vi "observacao_0MQ.vi"() -> ()   [LabVIEW 2012, in "Shared_160.lvlib"] (continued)
            # "MUDANÇA 10/8/2010 \nIncluídos:\n- Nome do instrumento\n- RA do telescópio"
            # "OBS: O Arquivo é inicialmente apagado para \nEvitar que fique corrompido!"
            # "Escreve arquivo com Dados para o Uso da Página do PDA"
            n1086 = global read "Global_Telescopio.vi" "Lista Instrumentos"() -> (w1420:string[])
            n1087 = global read "Global_Telescopio.vi" "Sideral Time"() -> (w1410:dbl)
            n1088 = global read "Global_Telescopio.vi" "PosAH"() -> (w1411:dbl)
            n1089 = global read "Global_Telescopio.vi" "Instrum"() -> (w1419:u16)
            n1090 = local read "DOMO_ENC"() -> (w1432:string)
            n1091 = local read "CUP_STAT"() -> (w1428:string)
            n1092 = local read "AH_STAT"() -> (w1430:string)
            n1093 = local read "Sideral time"() -> (w1439:string)
            n1094 = local read "AH_ENC"() -> (w1434:string)
            n1095 = local read "UT"() -> (w1438:string)
            n1096 = Subtract(x=w1410, y=w1411) -> (x-y=w1415:dbl)
            n1097 = Add(x=6.283185307179586, y=w1415) -> (x+y=w1414:dbl)
            n1098 = Less Than 0?(x=w1415) -> (x < 0?=w1412:bool)
            n1099 = call "Retira_tudo_depois_da_virgula.vi"("Entrada"=w1439) -> ("Saída"=w1436:string)
            n1100 = local read "TUBO_STAT"() -> (w1427:string)
            n1101 = Format Date/Time String(time format string (%c)="%H:%M:%S") -> (date/time string=w1422:string)  [unwired: 2 in]
            n1102 = local read "FOCO_ENC"() -> (w1431:string)
            n1103 = local read "DEC_STAT"() -> (w1429:string)
            n1104 = local read "DEC_ENC"() -> (w1433:string)
            n1105 = Select(t=w1414, s=w1412, f=w1415) -> (s? t:f=w1416:dbl)
            n1106 = Index Array(array=w1420, index=w1419) -> (element=w1421:string)
            n1107 = Format Date/Time String(time format string (%c)="%d/%m/%Y") -> (date/time string=w1423:string)  [unwired: 2 in]
            n1108 = call "Retira_tudo_depois_da_virgula.vi"("Entrada"=w1438) -> ("Saída"=w1435:string)
            n1109 = call <vilib>:"Trim Whitespace.vi"("string"=w1436) -> ("trimmed string"=w1426:string)  [unwired: 1 in]
            n1110 = call "rad_hms.vi"("TRUE=HORA\nFALSE=GRAU"=TRUE, "Radiano"=w1416) -> ("Hora/Graus Texto Decimal"=w1409:string)  [unwired: 3 in]
            n1111 = String To Path(string="C:\\TCS\\ARQUIVOS\\DadosTCSPD.txt") -> (path=w1440:path)
            n1112 = Concatenate Strings(w1423, w1418, w1422, w1418, w1435, w1418, w1426, w1418, w1434, w1418, w1433, w1418, w1432, w1418, w1431, w1418, w1430, w1418, w1429, w1418, w1428, w1418, w1427, w1418, w1421, w1418, w1409, w1418) -> (w1442:string)
            n1113 = case shown="True" "Case Constant\n(See Context Help) 2" {
              tunnel: [w1451 w1454] -> w1441
              tunnel: w1440 -> [w1451 w1453]
              frame False {
              }
              frame True {
                n1114 = Delete(path (use dialog)=w1453) -> (deleted path=w1454:path, error out=→"error out":errorcluster)  [unwired: 4 in, 1 out]
              }
            }
            n1115 = call <vilib>:"Open_Create_Replace File.vi"("function (open:0)"=T8."open or create", "file path"=w1441) -> ("error out"=w1446:errorcluster, "refnum"=w1449:refnum<file>)  [unwired: 6 in, 2 out]
            n1116 = Set File Position(refnum=w1449, from (0:start)=enum16{"start", "end", "current"}."start" ("pos mode (0:2)"), error in=w1446) -> (refnum out=w1408:refnum<file>, error out=w1407:errorcluster)  [unwired: 1 in]
            n1117 = Write to Binary File(file (use dialog)=w1408, data=w1442, error in=w1407, 5:FALSE ("prepend array or string size? (T)")) -> (refnum out=w1448:refnum<file>, error out=w1447:errorcluster)  [unwired: 2 in, 1 out]
            n1118 = Close File(refnum=w1448, error in=w1447) -> (error out=w1450:errorcluster)  [unwired: 1 out]
            n1119 = call <vilib>:"Simple Error Handler.vi"("error in (no error)"=w1450) -> ()  [unwired: 4 in, 5 out]
          }
          frame #15 {
            # "Página do PDA"
            # "http://192.168.1.1:1080/pdaWeb/"
            # "TRATAMENTO DO PDA"
            n1120 = stacked-sequence {
              frame #0 {
                # "MUDANÇA  3/9/2010 \nIncluído case abaixo e código de seu estado TRUE para apagar eventuais comandos do PDA enviados antes do TCSPD rodar."
                n1121 = First Call?() -> (First Call?: T/F=w1455:bool)
                n1122 = case shown="True" w1455 {
                  frame False {
                    # "MUDANÇA  4/9/2010 \nSubstituída a VI \"New Read PPC\" pela \"Trata PDA\" a qual evita que o telescópio seja apontado para regiões proibidas (inclinação excessiva)."
                    # "lê e interpreta o arquivo ppc.txt"
                    n1123 = call "Trata PDA.vi"() -> ()  [unwired: 2 in]
                  }
                  frame True {
                    n1124 = call "Find ppctxt.vi"() -> ("Existe ppc.txt?"=w1457:bool, "ppc.txt Path"=w1456:path)  [unwired: 1 in]
                    n1125 = case shown="True" w1457 {
                      tunnel: w1456 -> [_ w1458]
                      frame False {
                      }
                      frame True {
                        # "limpa o arquivo ppc.txt"
                        n1126 = call "Wipe file.vi"("ppc path"=w1458) -> ()  [unwired: 2 out]
                      }
                    }
                  }
                }
              }
              frame #1 {
                n1127 = case shown="False" "Case Constant\n(See Context Help) 3" {
                  frame False {
                  }
                  frame True {
                    # "MUDANÇA:\nÉ necesário \nsubstituir as variáveis simuladas pelas do Sistema"
                    # "Simula os dados sendo alterados pela\nmovimentação do sistema"
                    n1128 = call "Data Table.vi"() -> ()  [unwired: 1 in]
                  }
                }
              }
              frame #2 {
                n1129 = case shown="True" "Case Constant\n(See Context Help) 4" {
                  frame False {
                  }
                  frame True {
                    # "Lê o arquivo padrão para o equip/o\nselecionado pelo PDA e grava o\narquivo ppcDisplay.htm adequado"
                    n1130 = call "Update Frame.vi"() -> ("Timeout"=w1461:u32)  [unwired: 2 in, 3 out]
                    n1131 = Wait Until Next ms Multiple(millisecond multiple=w1461) -> ()  [unwired: 1 out]
                  }
                }
              }
            }
          }
        }
        n1132 = global read "Global_Telescopio.vi" "Flag-Rotator"() -> (w77:bool)
        n1133 = case shown="True" w77 {
          frame False {
          }
          frame True {
            n1134 = local write "Setup, Pointing & Guiding"(T2."ROTATOR" ("Setup, Pointing & Guiding")) -> ()
          }
        }
      }
      frame #2 {
        n1135 = case shown="\"UTILS \"" "Setup, Pointing & Guiding" {
          frame "POINTING", Default {
            n1136 = stacked-sequence {
              frame #0 {
                # "Clear Dados"
                n1137 = local read "ChkCalLocal"() -> (w1463:bool)
                n1138 = case shown="False" w1463 {
                  selector: w1463 -> [w1465 _]
                  frame False {
                    # "Para de Piscar/Blink\no botão"
                    n1139 = property on="ChkCalLocal" class="Bool (strict)"("Blinking"=w1465) -> ()  [unwired: 2 in, 2 out]
                  }
                  frame True {
                  }
                }
                n1140 = case shown="True" "BtPointObjClear" {
                  frame False {
                  }
                  frame True {
                    w1466 = ""
                    n1141 = local write "StrPointObjName"(w1466) -> ()
                    n1142 = local write "StrPointObjPMRA"(w1466) -> ()
                    n1143 = local write "StrPointObjPMDEC"(w1466) -> ()
                    n1144 = local write "StrPointObjRA"(w1466) -> ()
                    n1145 = local write "StrPointObjDEC"(w1466) -> ()
                    n1146 = local write "StrPointObjEpoch"(w1466) -> ()
                    n1147 = local write "StrPointTargetRA"(w1466) -> ()
                    n1148 = local write "StrPointTargetDEC"(w1466) -> ()
                  }
                }
              }
              frame #1 {
                w1473 = ""
                # "A forma como os mostradores da janela TARGET são carregados está indefinida.\nVamos colocar um botão SET ao lado do botão CLEAR na janela OBJECT.\nQuando o botão SET for pressionado, os mostradores da janela TARGET\nseriam calculados a partir dos valores da janela OBJECT."
                n1149 = local read "StrPointObjDEC"() -> (w1474:string)
                n1150 = local read "StrPointObjRA"() -> (w1475:string)
                n1151 = local read "StrPointObjPMDEC"() -> (w1467:string)
                n1152 = local read "StrPointObjPMRA"() -> (w1468:string)
                n1153 = Not Equal?(x=w1475, y=w1473) -> (x != y?=w1472:bool)
                n1154 = Not Equal?(x=w1474, y=w1473) -> (x != y?=w1471:bool)
                n1155 = local read "pressão atm"() -> (w1477:string)
                n1156 = local read "Temp amb"() -> (w1478:string)
                n1157 = local read "hum local"() -> (w1476:string)
                n1158 = And(x=w1472, y=w1471) -> (x .and. y?=w1469:bool)
                n1159 = And(x="BtPointPrecess", y=w1469) -> (x .and. y?=w1470:bool)
                n1160 = case shown="True" w1470 {
                  tunnel: w1475 -> [_ w1486]
                  tunnel: w1474 -> [_ w1485]
                  tunnel: w1478 -> [_ w1484]
                  tunnel: w1477 -> [_ w1483]
                  tunnel: w1476 -> [_ w1482]
                  tunnel: w1468 -> [_ w1481]
                  tunnel: w1467 -> [_ w1480]
                  frame False {
                  }
                  frame True {
                    n1161 = stacked-sequence {
                      tunnel: w1486 -> [w1520 _ _]
                      tunnel: w1485 -> [w1518 _ _]
                      tunnel: w1484 -> [w1528 _ _]
                      tunnel: w1483 -> [w1527 _ _]
                      tunnel: w1482 -> [w1526 _ _]
                      tunnel: w1481 -> [w1494 _ _]
                      tunnel: w1480 -> [w1493 _ _]
                      frame #0 {
                        # "PROCESSO PRECESSÃO"
                        # "MUDANÇA:\nVI Botao SET trocada por Botao Precess, eliminando entrada do Frame de coord. (Mean, Topo, Geo)"
                        n1162 = local read "ChkPointPrecessed"() -> (w1498:bool)
                        n1163 = call "Comma_to_Point.vi"("Lat_A"=w1518) -> ("Saída"=w1513:string)
                        n1164 = call "Comma_to_Point.vi"("Lat_A"=w1520) -> ("Saída"=w1516:string)
                        n1165 = call "hms_rad.vi"("True = hora"=FALSE, "Texto Graus"=w1513) -> ("radianos"=w1512:dbl)  [unwired: 3 in]
                        n1166 = call "hms_rad.vi"("True = hora"=TRUE, "Texto Graus"=w1516) -> ("radianos"=w1515:dbl)  [unwired: 3 in]
                        n1167 = call "Comma_to_Point.vi"("Lat_A"=w1527) -> ("Saída"=w1496:string)
                        n1168 = call "Comma_to_Point.vi"("Lat_A"=w1526) -> ("Saída"=w1495:string)
                        n1169 = call "Comma_to_Point.vi"("Lat_A"=w1528) -> ("Saída"=w1497:string)
                        n1170 = call "Arcsec to Rad_ String.vi"("VAR ARCSEC"=w1494) -> ("VAR RAD"=w1492:string)
                        n1171 = Number To Fractional String(use system decimal point (T)=FALSE, number=w1512, precision (6)=i16 9) -> (F-format string=w1501:string)  [unwired: 1 in]
                        n1172 = Number To Fractional String(use system decimal point (T)=FALSE, number=w1515, precision (6)=i16 9) -> (F-format string=w1502:string)  [unwired: 1 in]
                        n1173 = call "Arcsec to Rad_ String.vi"("VAR ARCSEC"=w1493) -> ("VAR RAD"=w1491:string)
                        n1174 = call "Botão Precess.vi"("AR"=w1502, "Precessed Coord."=w1498, "Dec"=w1501, "Temp local amb(K)"=w1497, "Pressao atm local (mB)"=w1496, "Hum rel local"=w1495, "Var RA"=w1492, "Var DEC"=w1491) -> ("RA"=w1530:dbl, "DEC"=w1487:dbl, "Hora Sideral (rad)"=w1529:dbl, "Dist. Zenital (rad)"=w1500:dbl, "Observed HA (radians)"=→"HA obs":dbl, "Massa de Ar"=w1499:dbl)  [unwired: 2 in]
                        "RA obs" <- w1530
                        "DEC obs" <- w1487
                        n1175 = local write "Zenital angle"(w1500) -> ()
                        n1176 = call "rad_hms.vi"("TRUE=HORA\nFALSE=GRAU"=FALSE ("TRUE=HORA\nFALSE=GRAU"), "Radiano"=w1487) -> ("Hora/Graus Texto Decimal"=w1508:string)  [unwired: 3 in]
                        n1177 = call "rad-graus.vi"("Radiano"=w1500) -> ("Graus"=w1525:dbl)
                        n1178 = Number To Fractional String(number=w1499, precision (6)=i16 3) -> (F-format string=→"Air Mass":string)  [unwired: 2 in]
                        n1179 = Number To Fractional String(number=w1525, precision (6)=i16 1) -> (F-format string=→"Zenital Angle":string)  [unwired: 2 in]
                        n1180 = call "rad_hms.vi"("TRUE=HORA\nFALSE=GRAU"=TRUE ("TRUE=HORA"), "Radiano"=w1530) -> ("Hora/Graus Texto Decimal"=w1510:string)  [unwired: 3 in]
                        n1181 = local write "StrPointTargetDEC"(w1508) -> ()
                        n1182 = local write "StrPointTargetRA"(w1510) -> ()
                        n1183 = disable-structure shown="Disabled" {
                          disable-tunnel: [w1534 _] -> _
                          disable-tunnel: w1530 -> [w1533 _]
                          disable-tunnel: w1529 -> [w1532 _]
                          disable-tunnel: w1487 -> [w1531 _]
                          frame Disabled {
                            n1184 = call "Hora_Limite.vi"("Asc Reta RA rad"=w1533, "Sideral Time rad"=w1532, "Declinação rad"=w1531) -> ("TO Tempo de Observação Horas"=w1534:dbl)  [unwired: 2 in]
                          }
                          frame Enabled {
                          }
                        }
                        n1185 = call "Novo_tempo_obs_inicial.vi"("TS"=w1529, "RA"=w1530, "DEC"=w1487) -> ("TO rad"=w1488:dbl)  [unwired: 7 in, 1 out]
                        n1186 = case shown="True" "TRUE=HORA\nFALSE=GRAU" {
                          frame False {
                          }
                          frame True {
                            # "Sincroniza hora do\nPC com GPS"
                            n1187 = call "About_Time.vi"() -> ()  [unwired: 1 in]
                          }
                        }
                        n1188 = call "rad_hms.vi"("TRUE=HORA\nFALSE=GRAU"=TRUE ("TRUE=HORA\nFALSE=GRAU"), "Radiano"=w1488) -> ("Hora/Graus Texto Decimal"=→"Tempo Obs":string)  [unwired: 3 in]
                      }
                      frame #1 {
                        # "Testa o ângulo zenital menor que 70º o led \"Working Area\" \naceso na cor verde se o ângulozenital menor que 70º e \nvermelho em caso cont rário."
                        n1189 = global read "Global_Telescopio.vi" "Piscar working area"() -> (w1541:bool)
                        n1190 = global read "Global_Telescopio.vi" "working area = VERDE"() -> (w1540:bool)
                        n1191 = global read "Global_Telescopio.vi" "ativar botão GO"() -> (w1538:bool)
                        n1192 = case shown="True" w1540 {
                          frame False {
                            # "False=Vermelho"
                            n1193 = local write "LedPointWorkArea"(FALSE ("LedPointWorkArea")) -> ()
                          }
                          frame True {
                            # "True=Verde"
                            "LedPointWorkArea" <- TRUE ("LedPointWorkArea")
                          }
                        }
                        n1194 = global write "Global_Telescopio.vi" "Botão GO = STOP"(FALSE ("Botão GO = STOP")) -> ()
                        n1195 = case shown="True" w1538 {
                          selector: w1538 -> [_ w1542]
                          frame False {
                          }
                          frame True {
                            n1196 = property on="BtTargetPoint" class="Bool"("Visible"=w1542) -> ()  [unwired: 2 in, 2 out]
                          }
                        }
                        n1197 = global write "Global_Telescopio.vi" "Piscar working area"(w1541) -> ()
                        n1198 = global read "Global_Telescopio.vi" "desativar botão GO"() -> (w1539:bool)
                        n1199 = case shown="True" w1539 {
                          selector: w1539 -> [_ w1544]
                          frame False {
                          }
                          frame True {
                            n1200 = Not(x=w1544) -> (.not. x?=w1543:bool)
                            n1201 = property on="BtTargetPoint" class="Bool"("Visible"=w1543) -> ()  [unwired: 2 in, 2 out]
                          }
                        }
                        n1202 = property on="LedPointWorkArea" class="Bool (strict)"("Visible"=TRUE ("Botão GO = STOP")) -> ()  [unwired: 2 in, 2 out]
                        n1203 = property on="LedPointing" class="Bool (strict)"("Visible"=FALSE) -> ()  [unwired: 2 in, 2 out]
                      }
                      frame #2 {
                        n1204 = global read "Global_Telescopio.vi" "CalDEC Local"() -> (w1552:dbl)
                        n1205 = global read "Global_Telescopio.vi" "CalAH Local"() -> (w1553:dbl)
                        n1206 = local read "ChkCalLocal"() -> (w1547:bool)
                        n1207 = Not Equal To 0?(x=w1553) -> (x != 0?=w1550:bool)
                        n1208 = Not Equal To 0?(x=w1552) -> (x != 0?=w1551:bool)
                        n1209 = Or(x=w1550, y=w1551) -> (x .or. y?=w1548:bool)
                        n1210 = And(x=w1547, y=w1548) -> (x .and. y?=w1549:bool)
                        n1211 = case shown="True" w1549 {
                          frame False {
                          }
                          frame True {
                            n1212 = local read "HA obs"() -> (w1573:dbl)
                            n1213 = local read "DEC obs"() -> (w1567:dbl)
                            n1214 = global read "Global_Telescopio.vi" "AH Zero Local"() -> (w1571:dbl)
                            n1215 = global read "Global_Telescopio.vi" "DEC Zero Local"() -> (w1566:dbl)
                            n1216 = global read "Global_Telescopio.vi" "Raio Máximo"() -> (w1555:dbl)
                            n1217 = Cosine(x=w1567) -> (cos(x)=w1572:dbl)
                            n1218 = Cosine(x=w1566) -> (cos(x)=w1570:dbl)
                            n1219 = Multiply(x=w1573, y=w1572) -> (x*y=w1569:dbl)
                            n1220 = Multiply(x=w1571, y=w1570) -> (x*y=w1568:dbl)
                            n1221 = Subtract(x=w1567, y=w1566) -> (x-y=w1562:dbl)
                            n1222 = Multiply(x=w1562, y=w1562) -> (x*y=w1565:dbl)
                            n1223 = Subtract(x=w1569, y=w1568) -> (x-y=w1561:dbl)
                            n1224 = Multiply(x=w1561, y=w1561) -> (x*y=w1563:dbl)
                            n1225 = Add(x=w1563, y=w1565) -> (x+y=w1564:dbl)
                            n1226 = Square Root(x=w1564) -> (sqrt(x)=w1560:dbl)
                            n1227 = Multiply(x=w1560, y=180.0) -> (x*y=w1558:dbl)
                            n1228 = Divide(x=w1558, y=3.141592653589793) -> (x/y=w1556:dbl)
                            n1229 = Greater?(x=w1556, y=w1555) -> (0:w1554:bool)
                            n1230 = property on="ChkCalLocal" class="Bool (strict)"("Blinking"=w1554) -> ()  [unwired: 2 in, 2 out]
                          }
                        }
                      }
                    }
                  }
                }
              }
              frame #2 {
                # "Clicando-se essa Tecla\nInicia-se o Apontamento"
                n1231 = local read "hum local"() -> (w1582:string)
                n1232 = local read "StrPointObjRA"() -> (w1584:string)
                n1233 = local read "StrPointObjDEC"() -> (w1583:string)
                n1234 = local read "StrPointObjPMDEC"() -> (w1575:string)
                n1235 = local read "pressão atm"() -> (w1576:string)
                n1236 = local read "StrPointObjPMRA"() -> (w1574:string)
                n1237 = local read "Temp amb"() -> (w1577:string)
                n1238 = control-ref of="BtTargetPoint"() -> (w1579:refnum<vi>)
                n1239 = property class="Bool"(reference=w1579) -> ("Boolean Text.Text"=w1580:string)  [unwired: 1 in, 2 out]
                n1240 = Equal?(x=w1580, y="POINT") -> (x = y?=w1578:bool)
                n1241 = case shown="True" "BtTargetPoint" {
                  tunnel: w1584 -> [_ w1590]
                  tunnel: w1583 -> [_ w1594]
                  tunnel: w1577 -> [_ w1591]
                  tunnel: w1576 -> [_ w1592]
                  tunnel: w1582 -> [_ w1593]
                  tunnel: w1578 -> [_ w1588]
                  tunnel: w1575 -> [_ w1587]
                  tunnel: w1574 -> [_ w1586]
                  frame False {
                  }
                  frame True {
                    n1242 = case shown="False" w1588 {
                      selector: w1588 -> [w1596 _]
                      tunnel: w1594 -> [_ w1626]
                      tunnel: w1593 -> [_ w1606]
                      tunnel: w1592 -> [_ w1605]
                      tunnel: w1591 -> [_ w1604]
                      tunnel: w1590 -> [_ w1625]
                      tunnel: w1587 -> [_ w1620]
                      tunnel: w1586 -> [_ w1621]
                      frame False {
                        w1597 = 0 ("estado")
                        # "Zera Máquina de Estado\nPelo Botão STOP"
                        n1243 = Not(x=w1596) -> (.not. x?=w1598:bool)
                        n1244 = local write "LedPointing"(w1596) -> ()
                        n1245 = global write "Global_Telescopio.vi" "Botão GO = STOP"(w1598) -> ()
                        n1246 = call "Stop.vi"() -> ()  [unwired: 1 in, 1 out]
                        n1247 = local write "statDEC"(w1597) -> ()
                        n1248 = local write "statAH"(w1597) -> ()
                        n1249 = local write "statCUP"(w1597) -> ()
                        "Flag Stop" <- TRUE ("Flag Stop")
                      }
                      frame True {
                        w1599 = ""
                        w1624 = FALSE ("use system decimal point (T)")
                        n1250 = call "Comma_to_Point.vi"("Lat_A"=w1625) -> ("Saída"=w1614:string)
                        n1251 = call "Comma_to_Point.vi"("Lat_A"=w1626) -> ("Saída"=w1615:string)
                        n1252 = call "Arcsec to Rad_ String.vi"("VAR ARCSEC"=w1621) -> ("VAR RAD"=w1602:string)
                        n1253 = call "hms_rad.vi"("True = hora"=TRUE, "Texto Graus"=w1614) -> ("radianos"=w1629:dbl)  [unwired: 3 in]
                        n1254 = call "hms_rad.vi"("True = hora"=FALSE, "Texto Graus"=w1615) -> ("radianos"=w1627:dbl)  [unwired: 3 in]
                        n1255 = call "Arcsec to Rad_ String.vi"("VAR ARCSEC"=w1620) -> ("VAR RAD"=w1603:string)
                        n1256 = local write "NAME"(w1599) -> ()
                        n1257 = local write "RA"(w1599) -> ()
                        n1258 = local write "DEC"(w1599) -> ()
                        n1259 = Number To Fractional String(use system decimal point (T)=w1624, number=w1629, precision (6)=i16 9) -> (F-format string=w1601:string)  [unwired: 1 in]
                        n1260 = Number To Fractional String(use system decimal point (T)=w1624, number=w1627, precision (6)=i16 9) -> (F-format string=w1600:string)  [unwired: 1 in]
                        n1261 = Concatenate Strings("Apontamento:" ("string"), "RA= " ("string"), w1614, " " ("string"), "DEC= " ("string"), w1615) -> ()  [unwired: 1 out]
                        n1262 = call "PrecessaoCorrigida.vi"("Coordenada do dia"="ChkPointPrecessed", "HabCorrModelo"="ChkModel", "UseLocalZero"="ChkCalLocal", "UseGlobalZero"="ChkCalGlobal", "RA"=w1601, "DEC"=w1600, "MovProprioRA"=w1602, "MovProprioDEC"=w1603, "Temp amb (K)"=w1604, "Press atm (mB)"=w1605, "Humid relat"=w1606) -> ("Estado"=w1609:i32, "RA"=w1608:dbl, "DEC"=w1607:dbl)  [unwired: 2 out]
                        n1263 = Equal To 0?(x=w1609) -> (x = 0?=w1622:bool)
                        n1264 = case shown="False" w1622 {
                          selector: w1622 -> [w1645 _]
                          tunnel: "ChkCalLocal" -> [w1657 _]
                          tunnel: "ChkCalGlobal" -> [w1656 _]
                          tunnel: w1600 -> [w1655 _]
                          tunnel: w1601 -> [w1654 _]
                          tunnel: w1603 -> [w1651 _]
                          tunnel: w1602 -> [w1650 _]
                          tunnel: w1609 -> [w1632 _]
                          tunnel: w1608 -> [w1653 _]
                          tunnel: w1607 -> [w1652 _]
                          tunnel: "ChkPointPrecessed" -> [w1648 _]
                          frame False {
                            w1635 = FALSE ("Coude")
                            w1636 = FALSE ("WeakSel")
                            w1637 = T5."Enabled" ("Disabled")
                            w1638 = TRUE ("MOUNT")
                            w1649 = 0 ("M_AH")
                            w1646 = TRUE
                            # "ABAS DE CONTROLE"
                            # "MUDANÇA:\nIncluído CASE"
                            # "Seta máquinas de\nestado aba ÚTILS"
                            n1265 = global write "Global_Telescopio.vi" "CoordDia"(w1648) -> ()
                            n1266 = global write "Global_Telescopio.vi" "CalGlobal"(w1656) -> ()
                            n1267 = global write "Global_Telescopio.vi" "CalLocal"(w1657) -> ()
                            n1268 = call "Envia LOG.vi"() -> ()  [unwired: 8 in, 2 out]
                            n1269 = global write "Global_Telescopio.vi" "TargetRA"(w1653) -> ()
                            n1270 = global write "Global_Telescopio.vi" "TargetDEC"(w1652) -> ()
                            n1271 = local write "statAH"(w1632) -> ()
                            n1272 = property on="LedPointWorkArea" class="Bool (strict)"("Visible"=FALSE ("Botão GO = STOP")) -> ()  [unwired: 2 in, 2 out]
                            n1273 = local write "statDEC"(w1632) -> ()
                            n1274 = global write "Global_Telescopio.vi" "ObjCentrado"(w1645) -> ()
                            n1275 = local write "RA on Target"(w1645) -> ()
                            n1276 = local write "DEC on Target"(w1645) -> ()
                            n1277 = local write "Dome on Target"(w1645) -> ()
                            n1278 = local read "ChkDomeEnable"() -> (w1644:bool)
                            n1279 = local write "M_AH"(w1649) -> ()
                            n1280 = local write "M_DEC"(w1649) -> ()
                            n1281 = local write "M_CUP"(w1649) -> ()
                            n1282 = case shown="True" w1644 {
                              selector: w1644 -> [w1678 _]
                              tunnel: w1632 -> [_ w1680]
                              tunnel: [0 ("Estado") w1680] -> w1643
                              tunnel: [u8 2 ("Disabled") u8 0 ("Disabled")] -> w1642
                              frame False {
                                n1283 = local write "DOME"(w1678) -> ()
                              }
                              frame True {
                              }
                            }
                            n1284 = Tick Count (ms)() -> (millisecond timer value=w1640:u32)
                            n1285 = Add(x=w1640, y=u32 120000) -> (x+y=w1641:u32)
                            n1286 = local write "Tick Cupula"(w1641) -> ()
                            n1287 = local write "GUIDER"(w1638) -> ()
                            n1288 = local write "MOUNT"(w1638) -> ()
                            n1289 = property on="LedPointing" class="Bool (strict)"("Visible"=w1646) -> ()  [unwired: 2 in, 2 out]
                            n1290 = local write "statCUP"(w1643) -> ()
                            n1291 = property on="DOME" class="Bool (strict)"("Disabled"=w1642) -> ()  [unwired: 2 in, 2 out]
                            n1292 = stacked-sequence {
                              frame #0 {
                                n1293 = local read "StrPointObjName"() -> (w1658:string)
                                n1294 = local read "StrPointObjRA"() -> (w1659:string)
                                n1295 = local read "StrPointObjDEC"() -> (w1660:string)
                                n1296 = global write "Global_Telescopio.vi" "RA AUX"(w1659) -> ()
                                n1297 = global write "Global_Telescopio.vi" "DEC AUX"(w1660) -> ()
                                n1298 = global write "Global_Telescopio.vi" "NAME OBJETO AUX"(w1658) -> ()
                              }
                              frame #1 {
                                w1662 = u16 4 items=["ZERO", "AH", "DEC", "TUBO", "CUP"] ("Controlador")
                                n1299 = call "Monta Comando.vi"("Comando"="DESLIGAR", "Dispositivo"="FLAT_WEAK", "Controlador"=w1662) -> ()  [unwired: 4 in, 3 out]
                              }
                              frame #2 {
                                w1665 = u16 4 items=["ZERO", "AH", "DEC", "TUBO", "CUP"] ("Controlador")
                                n1300 = call "Monta Comando.vi"("Comando"="DESLIGAR", "Dispositivo"="FLAT_LO", "Controlador"=w1665) -> ()  [unwired: 4 in, 3 out]
                              }
                              frame #3 {
                                w1668 = u16 4 items=["ZERO", "AH", "DEC", "TUBO", "CUP"] ("Controlador")
                                n1301 = call "Monta Comando.vi"("Comando"="DESLIGAR", "Dispositivo"="FLAT_HI", "Controlador"=w1668) -> ()  [unwired: 4 in, 3 out]
                              }
                              frame #4 {
                                w1670 = u16 4 items=["ZERO", "AH", "DEC", "TUBO", "CUP"] ("Controlador")
                                n1302 = call "Monta Comando.vi"("Comando"="DESLIGAR", "Dispositivo"="FLAT_COUDE", "Controlador"=w1670) -> ()  [unwired: 4 in, 3 out]
                              }
                              frame #5 {
                                w1673 = u16 4 items=["ZERO", "AH", "DEC", "TUBO", "CUP"] ("Controlador")
                                n1303 = call "Monta Comando.vi"("Comando"="LIGAR", "Dispositivo"="LAMP_CAM", "Controlador"=w1673) -> ()  [unwired: 4 in, 3 out]
                              }
                              frame #6 {
                                n1304 = call "Log_Apontamento.vi"() -> ()  [unwired: 12 in]
                              }
                            }
                            n1305 = local write "DOME"(FALSE ("WeakSel")) -> ()
                            n1306 = local write "WeakSel"(w1636) -> ()
                            n1307 = local write "MediumSel"(w1636) -> ()
                            n1308 = local write "StrongSel"(w1636) -> ()
                            n1309 = local write "CoudeSel"(w1636) -> ()
                            n1310 = local write "Coude"(w1635) -> ()
                            n1311 = local write "Weak"(w1635) -> ()
                            n1312 = local write "Medium"(w1635) -> ()
                            n1313 = local write "Strong"(w1635) -> ()
                            n1314 = property on="Medium" class="Bool (strict)"("Disabled"=w1637) -> ()  [unwired: 2 in, 2 out]
                            n1315 = property on="Strong" class="Bool (strict)"("Disabled"=w1637) -> ()  [unwired: 2 in, 2 out]
                            n1316 = property on="Coude" class="Bool (strict)"("DisabledEnum"=w1637) -> ()  [unwired: 2 in, 2 out]
                            n1317 = property on="Weak" class="Bool (strict)"("Disabled"=w1637) -> ()  [unwired: 2 in, 2 out]
                            "MeanDEC" <- w1655
                            "MeanRA" <- w1654
                            "LedPointing" <- w1646
                            "PM_DEC" <- w1651
                            "PM_RA" <- w1650
                            "Apontou" <- TRUE ("WeakSel")
                          }
                          frame True {
                          }
                        }
                      }
                    }
                    n1318 = property on="Delete Calagem" class="Bool"("Disabled"=u8 0) -> ()  [unwired: 2 in, 2 out]
                  }
                }
              }
              frame #3 {
                # "e o led \"Working Area\" aceso na cor verde se o ângulo\nzenital menor que 70º e vermelho em caso cont rário.\nO botão GO ao ser clicado dispara o apontamento virtual do telescópio. Caso esse\nbotão seja pressionado enquanto o led \"Working Area\" est iver vermelho, este deve\npiscar 3 vezes e nada mais é executado. Caso cont rário, o nome do botão GO passa\npara CANCEL e o led \"Mount in Posit ion\" da janela STATUS INFORMATION deve ser\ndesligado, o que provocará a simulação do apontamento do telescópio (cf. item 4.3) .\nOs valores dos comandos \"Epoch\" , \"RA Proper Mot ion\" e \"DEC Proper Mot ion\" desse\nquadro devem ser ignorados na simulação."
                # "Habilita Cancela"
                # "Habilita Apontamento"
                n1319 = case shown="True" "Case Constant\n(See Context Help) 5" {
                  frame False {
                  }
                  frame True {
                    w1686 = TRUE ("Go aux")
                    w1687 = ""
                    n1320 = local write "DEC"(w1687) -> ()
                    n1321 = local write "RA"(w1687) -> ()
                    n1322 = local write "NAME"(w1687) -> ()
                    n1323 = control-ref of="BtTargetPoint"() -> (w1688:refnum<vi>)
                    n1324 = local write "LED MOUNT"(w1686) -> ()
                    n1325 = local write "MOUNT"(w1686) -> ()
                    n1326 = property class="Bool"(reference=w1688, "Boolean Text.Text"="STOP") -> ()  [unwired: 1 in, 2 out]
                  }
                }
                n1327 = case shown="True" "Case Constant\n(See Context Help) 6" {
                  frame False {
                  }
                  frame True {
                    w1683 = FALSE ("Go aux")
                    # "Seta nome para GO"
                    n1328 = local write "LED MOUNT"(w1683) -> ()
                    n1329 = local write "MOUNT"(w1683) -> ()
                    n1330 = control-ref of="BtTargetPoint"() -> (w1684:refnum<vi>)
                    n1331 = property class="Bool"(reference=w1684, "Boolean Text.Text"="POINT") -> ()  [unwired: 1 in, 2 out]
                  }
                }
              }
              frame #4 {
                # "Detecta Edição"
                # "os valores de RA e DEC devem assumir os valores da janela OBJECT da aba POINTING ao TÉRMINO do apontamento. Durante o apontamento devem ficar apagados. Como o campo MAG daquela janela não tem um valor correspondente na janela OBJECT, o campo MAG deve ficar em branco. Apenas quando as coordenadas da janela OBJECT da aba POINTING forem preenchidos a partir do botão SET COORD da aba LIST é que o campo MAG da janela TARGET assume o valor da coluna MAG da aba LIST. Colocar um flag interno (invisível para o usuário) para definir se o campo MAG deve ou não ser preenchido com o valor da aba LIST. Quando o botão SET COORD. fosse pressionado esse flag assumiria o valor verdadeiro e caso ocorresse edição dos valores da janela \nOBJECT da aba POINTING, esse flag assumiria o valor falso e o campo MAG da janela TARGET (entre os controles das abas e as imagens) ficaria vazio durante e após o apontamento"
                n1332 = local read "StrPointObjPMRA"() -> (w1703:string)
                n1333 = local read "StrPointObjPMDEC"() -> (w1702:string)
                n1334 = local read "StrPointObjName"() -> (w1710:string)
                n1335 = local read "AUX EDITA Name"() -> (w1709:string)
                n1336 = local read "StrPointObjEpoch"() -> (w1704:string)
                n1337 = local read "AUX EDITA PMDEC"() -> (w1701:string)
                n1338 = local read "StrPointObjRA"() -> (w1708:string)
                n1339 = local read "StrPointObjDEC"() -> (w1706:string)
                n1340 = local read "AUX EDITA EPOCH"() -> (w1699:string)
                n1341 = local read "AUX EDITA PMRA"() -> (w1700:string)
                n1342 = local read "AUX EDITA DEC"() -> (w1705:string)
                n1343 = local read "AUX EDITA RA"() -> (w1707:string)
                n1344 = Not Equal?(x=w1703, y=w1700) -> (x != y?=w1694:bool)
                n1345 = Not Equal?(x=w1710, y=w1709) -> (x != y?=w1698:bool)
                n1346 = Not Equal?(x=w1704, y=w1699) -> (x != y?=w1695:bool)
                n1347 = Not Equal?(x=w1702, y=w1701) -> (x != y?=w1693:bool)
                n1348 = Not Equal?(x=w1708, y=w1707) -> (x != y?=w1697:bool)
                n1349 = Not Equal?(x=w1706, y=w1705) -> (x != y?=w1696:bool)
                n1350 = Compound Arithmetic op=OR(w1698, w1697, w1696, w1695, w1694, w1693) -> (w1690:bool)
                n1351 = local read "FLAG SET COORD"() -> (w1691:bool)
                n1352 = And(x=w1690, y=w1691) -> (x .and. y?=w1692:bool)
                n1353 = case shown="True" w1692 {
                  frame False {
                  }
                  frame True {
                    # "Se houver edição o flag é resetado"
                    n1354 = local write "MAG"("") -> ()
                    "FLAG SET COORD" <- FALSE ("FLAG SET ACOORD")
                  }
                }
              }
            }
          }
          frame "HANDSET" {
            # "PROCESSO DISPLAY DESLOCAMENTO"
            n1355 = local read "AtualDEC"() -> (w1726:dbl)
            n1356 = global read "Global_Telescopio.vi" "Sideral Time"() -> (w1719:dbl)
            n1357 = global read "Global_Telescopio.vi" "PosAH"() -> (w1717:dbl)
            n1358 = Multiply(x="Velocity (arcsec/sec)", y=100.0) -> (x*y=w1734:dbl)
            n1359 = Cosine(x=w1726) -> (cos(x)=w1725:dbl)
            n1360 = Subtract(x=w1719, y=w1717) -> (x-y=w1718:dbl)
            n1361 = Absolute Value(x=w1725) -> (abs(x)=w1722:dbl)
            n1362 = Add(x=1e-10, y=w1722) -> (x+y=w1724:dbl)
            n1363 = local read "LatchDeslocRA"() -> (w1730:dbl)
            n1364 = local read "LatchDeslocDEC"() -> (w1729:dbl)
            n1365 = global read "Global_Telescopio.vi" "PosDEC"() -> (w1720:dbl)
            n1366 = event shown="[9] \"Calagem\": Value Change" {
              selector: _ -> [_ _ _ _ _ _ _ _ _ _ _]
              dyn-events: _ -> [_ _ _ _ _ _ _ _ _ _ _]
              timeout: 10 -> [_ _ _ _ _ _ _ _ _ _ _]
              tunnel: w1734 -> [_ w1747 w1755 w1763 _ _ _ _ _ _ w1866]
              tunnel: "Global" -> [_ _ _ _ _ _ _ _ w1808 w1828 _]
              tunnel: w1718 -> [_ _ _ _ w1766 _ _ _ _ w1826 _]
              tunnel: w1720 -> [_ _ _ _ _ w1767 _ _ _ w1827 _]
              tunnel: w1724 -> [_ _ _ _ _ _ w1768 w1786 _ _ _]
              event Timeout {
                n1367 = event-data() -> ()  [unwired: 1 in, 2 out]
              }
              event "Left HS": Value Change {
                w1744 = u8 0 ("Disabled")
                n1368 = event-data() -> ("NewVal"=w1743:bool)  [unwired: 1 in, 5 out]
                "MOV_IDX_AH" <- w1743
                n1369 = call "Tx handeset.vi"("CMD On"="left" ("Comando"), "CMD Off"="stoph" ("Comando"), "Estado do Botão"=w1743, "Velocity (arcsec/sec)"=w1747) -> ()  [unwired: 12 in]
                n1370 = Select(t=u8 2 ("Disabled"), s=FALSE, f=w1744) -> (s? t:f=w1745:u8)
                n1371 = property on="Delete Calagem" class="Bool"("Disabled"=w1744) -> ()  [unwired: 2 in, 2 out]
                n1372 = property on="Right HS" class="Bool (strict)"("Disabled"=w1745) -> ()  [unwired: 2 in, 2 out]
              }
              event "Down HS": Value Change {
                w1751 = u8 0 ("Disabled")
                n1373 = event-data() -> ("NewVal"=w1754:bool)  [unwired: 1 in, 5 out]
                "MOV_IDX_DEC" <- w1754
                n1374 = call "Tx handeset.vi"("CMD On"="down" ("Comando"), "CMD Off"="stopv" ("Comando"), "Estado do Botão"=w1754, "Velocity (arcsec/sec)"=w1755) -> ()  [unwired: 12 in]
                n1375 = Select(t=u8 2 ("Disabled"), s=FALSE, f=w1751) -> (s? t:f=w1752:u8)
                n1376 = property on="Delete Calagem" class="Bool"("Disabled"=w1751) -> ()  [unwired: 2 in, 2 out]
                n1377 = property on="Up HS" class="Bool (strict)"("Disabled"=w1752) -> ()  [unwired: 2 in, 2 out]
              }
              event "Right HS": Value Change {
                w1760 = u8 0 ("Disabled")
                n1378 = event-data() -> ("NewVal"=w1759:bool)  [unwired: 1 in, 5 out]
                n1379 = call "Tx handeset.vi"("CMD On"="right" ("Comando"), "CMD Off"="stoph" ("Comando"), "Estado do Botão"=w1759, "Velocity (arcsec/sec)"=w1763) -> ()  [unwired: 12 in]
                n1380 = local write "MOV_IDX_AH"(w1759) -> ()
                n1381 = Select(t=u8 2 ("Disabled"), s=FALSE, f=w1760) -> (s? t:f=w1761:u8)
                n1382 = property on="Delete Calagem" class="Bool"("Disabled"=w1760) -> ()  [unwired: 2 in, 2 out]
                n1383 = property on="Left HS" class="Bool (strict)"("Disabled"=w1761) -> ()  [unwired: 2 in, 2 out]
              }
              event "ClearDeslocRA": Value Change {
                n1384 = event-data() -> ()  [unwired: 1 in, 6 out]
                "LatchDeslocRA" <- w1766
              }
              event "ClearDeslocDEC": Value Change {
                n1385 = event-data() -> ()  [unwired: 1 in, 6 out]
                "LatchDeslocDEC" <- w1767
              }
              event "BtPrecCentrar": Value Change {
                # "PROCESSO OFFSET"
                n1386 = event-data() -> ()  [unwired: 1 in, 6 out]
                n1387 = stacked-sequence {
                  tunnel: w1768 -> [_ w1777]
                  frame #0 {
                    n1388 = local read "Offset DEC"() -> (w1769:dbl)
                    n1389 = Negate(x=w1769) -> (-x=w1770:dbl)
                    n1390 = Equal To 0?(x=w1769) -> (x = 0?=w1771:bool)
                    n1391 = case shown="False" w1771 {
                      tunnel: w1770 -> [w1772 _]
                      frame False {
                        n1392 = call "Conversao Ms to Hora texto.vi"("TRUE=HORA\nFALSE=GRAU"=FALSE ("TRUE=HORA\nFALSE=GRAU"), "PrecDEC"=w1772) -> ("Hora/Graus Texto Decimal"=w1774:string)
                        n1393 = call "Tx handeset.vi"("CMD On"="goDEC", "Set Point"=w1774, "Estado do Botão"=TRUE ("TRUE=HORA\nFALSE=GRAU")) -> ()  [unwired: 13 in]
                      }
                      frame True {
                      }
                    }
                  }
                  frame #1 {
                    # "PROCESSO MOVE TELESCÓPIO"
                    n1394 = local read "Offset RA"() -> (w1778:dbl)
                    n1395 = Equal To 0?(x=w1778) -> (x = 0?=w1779:bool)
                    n1396 = case shown="False" w1779 {
                      tunnel: w1778 -> [w1781 _]
                      tunnel: w1777 -> [w1780 _]
                      frame False {
                        w1783 = TRUE ("TRUE=HORA\nFALSE=GRAU")
                        # "AH tem sentido\ncontrário de RA"
                        n1397 = Divide(x=w1781, y=w1780) -> (x/y=w1782:dbl)
                        n1398 = call "Conversao Ms to Hora texto.vi"("TRUE=HORA\nFALSE=GRAU"=w1783, "PrecDEC"=w1782) -> ("Hora/Graus Texto Decimal"=w1784:string)
                        n1399 = call "Tx handeset.vi"("CMD On"="goRA", "Set Point"=w1784, "Estado do Botão"=w1783) -> ()  [unwired: 13 in]
                      }
                      frame True {
                      }
                    }
                  }
                }
              }
              event "BtPrecGO": Value Change {
                # "PROCESSO OFFSET"
                n1400 = event-data() -> ("NewVal"=w1788:bool)  [unwired: 1 in, 5 out]
                n1401 = property on="Delete Calagem" class="Bool"("Disabled"=u8 2) -> ()  [unwired: 2 in, 2 out]
                n1402 = case shown="True" w1788 {
                  tunnel: w1786 -> [_ w1789]
                  frame False {
                  }
                  frame True {
                    # "PROCESSO MOVE TELESCÓPIO"
                    n1403 = stacked-sequence {
                      tunnel: w1789 -> [_ w1797]
                      frame #0 {
                        n1404 = Not Equal To 0?(x="PreciseOffsetDEC") -> (x != 0?=w1791:bool)
                        n1405 = case shown="True" w1791 {
                          tunnel: "PreciseOffsetDEC" -> [_ w1792]
                          frame False {
                          }
                          frame True {
                            n1406 = call "Conversao Ms to Hora texto.vi"("TRUE=HORA\nFALSE=GRAU"=FALSE ("TRUE=HORA\nFALSE=GRAU"), "PrecDEC"=w1792) -> ("Hora/Graus Texto Decimal"=w1794:string)
                            n1407 = call "Tx handeset.vi"("CMD On"="goDEC", "Set Point"=w1794, "Estado do Botão"=TRUE ("TRUE=HORA\nFALSE=GRAU")) -> ()  [unwired: 13 in]
                          }
                        }
                      }
                      frame #1 {
                        n1408 = Not Equal To 0?(x="PreciseOffsetRA") -> (x != 0?=w1800:bool)
                        n1409 = Negate(x="PreciseOffsetRA") -> (-x=w1799:dbl)
                        n1410 = case shown="True" w1800 {
                          tunnel: w1799 -> [_ w1802]
                          tunnel: w1797 -> [_ w1801]
                          frame False {
                          }
                          frame True {
                            n1411 = Divide(x=w1802, y=w1801) -> (x/y=w1803:dbl)
                            n1412 = call "Conversao Ms to Hora texto.vi"("TRUE=HORA\nFALSE=GRAU"=TRUE ("TRUE=HORA\nFALSE=GRAU"), "PrecDEC"=w1803) -> ("Hora/Graus Texto Decimal"=w1805:string)
                            n1413 = call "Tx handeset.vi"("CMD On"="goRA", "Set Point"=w1805, "Estado do Botão"=TRUE ("TRUE=HORA\nFALSE=GRAU")) -> ()  [unwired: 13 in]
                          }
                        }
                      }
                    }
                  }
                }
              }
              event "Delete Calagem": Value Change {
                n1414 = event-data() -> ()  [unwired: 1 in, 6 out]
                n1415 = case shown="True" w1808 {
                  tunnel: 0.0 ("Calagem DEC Rel") -> [w1810 w1811]
                  frame False {
                    # "Local"
                    n1416 = global write "Global_Telescopio.vi" "CalAH Local"(w1810) -> ()
                    n1417 = global write "Global_Telescopio.vi" "CalDEC Local"(w1810) -> ()
                  }
                  frame True {
                    # "Global"
                    n1418 = global write "Global_Telescopio.vi" "Calagem AH"(w1811) -> ()
                    n1419 = global write "Global_Telescopio.vi" "Calagem DEC"(w1811) -> ()
                  }
                }
              }
              event "Calagem": Value Change {
                # "PROCESSO CALAGEM"
                n1420 = event-data() -> ()  [unwired: 1 in, 6 out]
                n1421 = local read "ChkModel"() -> (w1817:bool)
                n1422 = local read "Temp amb"() -> (w1821:string)
                n1423 = local read "hum local"() -> (w1823:string)
                n1424 = local read "MeanDEC"() -> (w1814:string)
                n1425 = local read "MeanRA"() -> (w1818:string)
                n1426 = local read "PM_RA"() -> (w1819:string)
                n1427 = local read "PM_DEC"() -> (w1820:string)
                n1428 = local read "pressão atm"() -> (w1822:string)
                n1429 = global read "Global_Telescopio.vi" "CalGlobal"() -> (w1815:bool)
                n1430 = global read "Global_Telescopio.vi" "CalLocal"() -> (w1816:bool)
                n1431 = global read "Global_Telescopio.vi" "CoordDia"() -> (w1813:bool)
                n1432 = call "PrecessaoCorrigida.vi"("Coordenada do dia"=w1813, "HabCorrModelo"=w1817, "UseLocalZero"=w1816, "UseGlobalZero"=w1815, "RA"=w1818, "DEC"=w1814, "MovProprioRA"=w1819, "MovProprioDEC"=w1820, "Temp amb (K)"=w1821, "Press atm (mB)"=w1822, "Humid relat"=w1823) -> ("RA"=w1825:dbl, "DEC"=w1824:dbl, "AH"=w1812:dbl)  [unwired: 2 out]
                n1433 = case shown="False" w1828 {
                  tunnel: w1825 -> [w1838 w1841]
                  tunnel: w1824 -> [w1830 w1843]
                  tunnel: w1827 -> [w1837 w1844]
                  tunnel: w1826 -> [w1839 w1842]
                  tunnel: w1812 -> [w1829 _]
                  frame False {
                    # "Local"
                    n1434 = Subtract(x=w1839, y=w1838) -> (x-y=w1840:dbl)
                    n1435 = Subtract(x=w1837, y=w1830) -> (x-y=w1834:dbl)
                    n1436 = global read "Global_Telescopio.vi" "CalAH Local"() -> (w1833:dbl)
                    n1437 = global read "Global_Telescopio.vi" "CalDEC Local"() -> (w1835:dbl)
                    n1438 = global write "Global_Telescopio.vi" "AH Zero Local"(w1829) -> ()
                    n1439 = global write "Global_Telescopio.vi" "DEC Zero Local"(w1830) -> ()
                    n1440 = Negate(x=w1840) -> (-x=w1836:dbl)
                    n1441 = Add(x=w1836, y=w1833) -> (x+y=w1832:dbl)
                    n1442 = Add(x=w1834, y=w1835) -> (x+y=w1831:dbl)
                    n1443 = global write "Global_Telescopio.vi" "CalAH Local"(w1832) -> ()
                    n1444 = global write "Global_Telescopio.vi" "CalDEC Local"(w1831) -> ()
                  }
                  frame True {
                    # "Global"
                    n1445 = stacked-sequence {
                      tunnel: w1844 -> [w1854 _ _]
                      tunnel: w1843 -> [w1853 _ _]
                      tunnel: w1842 -> [w1849 _ _]
                      tunnel: w1841 -> [w1848 _ _]
                      frame #0 {
                        w1845 = 0.0 ("CalAH Local")
                        n1446 = Subtract(x=w1849, y=w1848) -> (x-y=w1847:dbl)
                        n1447 = Subtract(x=w1854, y=w1853) -> (x-y=w1855:dbl)
                        n1448 = global read "Global_Telescopio.vi" "Calagem AH"() -> (w1852:dbl)
                        n1449 = global read "Global_Telescopio.vi" "Calagem DEC"() -> (w1857:dbl)
                        n1450 = Negate(x=w1847) -> (-x=w1850:dbl)
                        n1451 = local write "Processa Centragem"(TRUE) -> ()
                        n1452 = Add(x=w1850, y=w1852) -> (x+y=w1851:dbl)
                        n1453 = Add(x=w1855, y=w1857) -> (x+y=w1856:dbl)
                        n1454 = global write "Global_Telescopio.vi" "Calagem AH"(w1851) -> ()
                        n1455 = global write "Global_Telescopio.vi" "CalAH Local"(w1845) -> ()
                        n1456 = global write "Global_Telescopio.vi" "CalDEC Local"(w1845) -> ()
                        n1457 = global write "Global_Telescopio.vi" "Calagem DEC"(w1856) -> ()
                      }
                      frame #1 {
                        # "25/10/2012 - Sempre que o usuario faz uma \ncalagem global, o valor da calagem e'  salva \nautomaticamente em GLOBAIS_CALAGEM.DAT"
                        n1458 = call "Salva_Calagem_Global.vi"() -> ()  [unwired: 1 in]
                      }
                      frame #2 {
                        # "Salva no Logo valor \ndo deslocamento da \ncalagem global"
                        n1459 = local read "DeslocDEC"() -> (w1858:dbl)
                        n1460 = local read "DeslocRA"() -> (w1859:dbl)
                        n1461 = call "Log_Calagem.vi"("Desloc DEC"=w1858, "Desloc RA"=w1859, "File Name"="LOG_COMANDOS.TXT") -> ()  [unwired: 3 in]
                      }
                    }
                  }
                }
              }
              event "Up HS": Value Change {
                w1863 = u8 0 ("Disabled")
                n1462 = event-data() -> ("NewVal"=w1862:bool)  [unwired: 1 in, 5 out]
                n1463 = call "Tx handeset.vi"("CMD On"="up" ("Comando"), "CMD Off"="stopv" ("Comando"), "Estado do Botão"=w1862, "Velocity (arcsec/sec)"=w1866) -> ()  [unwired: 12 in]
                n1464 = local write "MOV_IDX_DEC"(w1862) -> ()
                n1465 = property on="Delete Calagem" class="Bool"("Disabled"=w1863) -> ()  [unwired: 2 in, 2 out]
                n1466 = Select(t=u8 2 ("Disabled"), s=FALSE, f=w1863) -> (s? t:f=w1864:u8)
                n1467 = property on="Down HS" class="Bool (strict)"("Disabled"=w1864) -> ()  [unwired: 2 in, 2 out]
              }
            }
            n1468 = Subtract(x=w1718, y=w1730) -> (x-y=w1727:dbl)
            n1469 = Subtract(x=w1720, y=w1729) -> (x-y=w1731:dbl)
            n1470 = Multiply(x=w1727, y=w1724) -> (x*y=w1728:dbl)
            n1471 = global read "Global_Telescopio.vi" "ObjCentrado"() -> (w1721:bool)
            n1472 = call "Rad to Arcsec.vi"("Radiano"=w1728) -> ("Arcsec"=w1714:dbl)
            n1473 = call "Rad to Arcsec.vi"("Radiano"=w1731) -> ("Arcsec"=w1713:dbl)
            n1474 = case shown="False" w1721 {
              tunnel: [w1737 w1739] -> w1716
              tunnel: [w1737 w1740] -> w1715
              tunnel: w1714 -> [_ w1740]
              tunnel: w1713 -> [_ w1739]
              frame False {
                w1737 = 0.0 ("DeslocRA")
                n1475 = property on="Calagem" class="Bool"("Disabled"=u8 2) -> ()  [unwired: 2 in, 2 out]
              }
              frame True {
                n1476 = property on="Calagem" class="Bool"("Disabled"=u8 0) -> ()  [unwired: 2 in, 2 out]
              }
            }
            "DeslocRA" <- w1715
            "DeslocDEC" <- w1716
          }
          frame "GUIDER" {
            w1879 = 1 ("lower limit")
            w1880 = 400 ("upper limit")
            # "PROCESSO VARIABLE TRACKING"
            n1477 = call "Borda Subida.vi"("Entrada"="VARIABLE \nTRACKING") -> ("Boolean"=w1885:bool)  [unwired: 4 in]
            n1478 = call "Borda.vi"("Entrada"="VARIABLE \nTRACKING") -> ("Boolean"=w1884:bool)  [unwired: 4 in]
            n1479 = case shown="True" w1884 {
              frame False {
              }
              frame True {
                w1940 = "0" ("Set Point")
                w1946 = u16 2 items=["ZERO", "AH", "DEC", "TUBO", "CUP"] ("Controlador")
                w1943 = u16 1 items=["ZERO", "AH", "DEC", "TUBO", "CUP"] ("Controlador")
                # "Enviando ZERO o controlador para o movimento"
                n1480 = call "Monta Comando.vi"("Set Point"=w1940, "Comando"="GIRAR_VEL", "Dispositivo"="EIXO" ("Comando"), "Controlador"=w1943) -> ()  [unwired: 3 in, 3 out]
                n1481 = call "Monta Comando.vi"("Set Point"=w1940, "Comando"="GIRAR_VEL", "Dispositivo"="EIXO" ("Comando"), "Controlador"=w1946) -> ()  [unwired: 3 in, 3 out]
              }
            }
            n1482 = case shown="True" w1885 {
              frame False {
              }
              frame True {
                w1957 = u16 2 items=["ZERO", "AH", "DEC", "TUBO", "CUP"] ("Controlador")
                w1954 = u16 1 items=["ZERO", "AH", "DEC", "TUBO", "CUP"] ("Controlador")
                # "Enviar esses Valores \npara os controladores"
                n1483 = property on="Calagem" class="Bool"("Disabled"=u8 2) -> ()  [unwired: 2 in, 2 out]
                n1484 = Number To Decimal String(number="RA  RATE") -> (decimal integer string=w1950:string)  [unwired: 1 in]
                n1485 = Number To Decimal String(number="DEC RATE") -> (decimal integer string=w1948:string)  [unwired: 1 in]
                n1486 = call "Monta Comando.vi"("Set Point"=w1950, "Comando"="GIRAR_VEL", "Dispositivo"="EIXO" ("Comando"), "Controlador"=w1954) -> ()  [unwired: 3 in, 3 out]
                n1487 = call "Monta Comando.vi"("Set Point"=w1948, "Comando"="GIRAR_VEL", "Dispositivo"="EIXO" ("Comando"), "Controlador"=w1957) -> ()  [unwired: 3 in, 3 out]
              }
            }
            n1488 = case shown="True" "ClearDEC" {
              frame False {
              }
              frame True {
                n1489 = local write "DEC RATE"(0 ("RA  RATE")) -> ()
              }
            }
            n1490 = case shown="True" "ClearRA" {
              frame False {
              }
              frame True {
                n1491 = local write "RA  RATE"(0 ("RA  RATE")) -> ()
              }
            }
            n1492 = In Range and Coerce(upper limit=w1880, x="X STAR", lower limit=w1879) -> (In Range?=w1876:bool)  [unwired: 1 out]
            n1493 = In Range and Coerce(upper limit=w1880, x="Y STAR", lower limit=w1879) -> (In Range?=w1877:bool)  [unwired: 1 out]
            n1494 = In Range and Coerce(upper limit=w1880, x="X CENTER", lower limit=w1879) -> (In Range?=w1875:bool)  [unwired: 1 out]
            n1495 = In Range and Coerce(upper limit=w1880, x="Y CENTER", lower limit=w1879) -> (In Range?=w1874:bool)  [unwired: 1 out]
            n1496 = Compound Arithmetic op=AND(w1876, w1877, w1875, w1874, "XY CENTER") -> (w1878:bool)
            n1497 = case shown="True" w1878 {
              tunnel: "X STAR" -> [_ w1921]
              tunnel: "X CENTER" -> [_ w1920]
              tunnel: "Y STAR" -> [_ w1919]
              tunnel: "Y CENTER" -> [_ w1918]
              frame False {
              }
              frame True {
                # "MUDANÇA: IMPLEMENTADO MOV. XY DO GUIDER EM \n20-05-2011, MAS AINDA NÃO FOI TESTADO..."
                # "rad"
                # "Ativa o envio comando de deslocamento ao controlador"
                n1498 = global read "Global_Telescopio.vi" "guide_ang"() -> (w1909:string)
                n1499 = global read "Global_Telescopio.vi" "guide_nor"() -> (w1910:string)
                n1500 = global read "Global_Telescopio.vi" "guide_cas"() -> (w1917:string)
                n1501 = Subtract(x=w1921, y=w1920) -> (x-y=w1915:i32)
                n1502 = Subtract(x=w1919, y=w1918) -> (x-y=w1914:i32)
                n1503 = global read "Global_Telescopio.vi" "guide_esp"() -> (w1912:string)
                n1504 = To Double Precision Float(number=w1915) -> (double precision float=w1892:dbl)
                n1505 = To Double Precision Float(number=w1914) -> (double precision float=w1893:dbl)
                n1506 = Equal?(x=w1917, y="S") -> (x = y?=w1907:bool)
                n1507 = case shown="True" w1907 {
                  tunnel: w1910 -> [_ w1937]
                  tunnel: w1909 -> [_ w1934]
                  tunnel: [w1930 w1931] -> w1906
                  frame False {
                    # "Foco Coudé"
                    n1508 = call "AnguloFenda.vi"() -> ("AngFenda"=w1930:dbl)  [unwired: 3 in]
                  }
                  frame True {
                    # "Foco Cassegrain"
                    n1509 = Fract/Exp String To Number(use system decimal point (T)=FALSE, string=w1937) -> (number=w1932:dbl)  [unwired: 2 in, 1 out]
                    n1510 = Fract/Exp String To Number(use system decimal point (T)=FALSE, string=w1934) -> (number=w1933:dbl)  [unwired: 2 in, 1 out]
                    n1511 = Add(x=w1933, y=w1932) -> (x+y=w1931:dbl)
                  }
                }
                n1512 = Equal?(x=w1912, y="S") -> (x = y?=w1897:bool)
                n1513 = global write "Global_Telescopio.vi" "Correção Guider"("Habilita Movimento") -> ()
